vi "Run - TDMS Logging (SubVI).vi"(8 "error in (no error)":errorcluster, 10 "Cluster":T1={"Test Plan"=[], "PlanRow"=0, "Device Name"=[], "Timeout"=0, "Start?"=FALSE, "Pause?"=FALSE, "IP Address"=[], "LogRow"=0, "Logtype"=0, "Log Elapse"=0.0, "Data"={"Station"="", "Sample ID"="", "Job No"="", "Job Description"="", "Path"=path "", "Delay"=timestamp(-28800 s since 1904-01-01), "Square"=FALSE, "Test Type"=0, "Speciment No"="", "Depth"="", "Height"="", "Diameter/Length"="", "Weight"=""}, "Stop log?"=FALSE, "tdms"=refnum, "Sensor Data"=[], "Start time"=timestamp(0 s since 1904-01-01), "Prev Log Elapse"=0, "Plot"=0, "X-Axis"=[], "Y-Axis"=[], "XY"=[], "End Stage?"=FALSE, "1run"=FALSE, "Condition"=[], "Start Con"=FALSE, "Log Con"=FALSE, "Stop Con"=FALSE, "Start Elapse"=0.0, "Start Load"=0.0, "Motor"=0, "StartRow"=0, "number log"=0, "Dir"=FALSE, "Start time test"=timestamp(0 s since 1904-01-01), "Auto"=FALSE, "Check return?"=FALSE, "Inv"={"M"=[], "Bool"=[]}, "tdms temp"=refnum, "Zero?"=FALSE, "Graph timer"=0.0, "Square"=FALSE, "Plot Timer"=0.0, "1st Run"=FALSE, "TDMS Path"=path "", "MaxLoad"=0.0, "Log Timer"=[], "Test Type"=0, "Log Sensor"=[], "Save?"=FALSE, "1st Log"=FALSE, "Y-Axis 2"=[], "On Y-Axis 2"=FALSE, "Decimal"=[], "Init"={"PWP"=0.0, "Load"=0.0, "Volume"=0.0, "Disp"=0.0, "CP"=0.0, "Vol In"=0.0, "Vol Out"=0.0}, "Calc"={"TS"={"Change PWP"=0.0, "Change Vol"=0.0, "Axial Load"=0.0, "CiL"=0.0, "Deviator"=0.0, "Axial Strain"=0.0}, "TUU"={"Change PWP"=0.0, "Axial Load"=0.0, "CiL"=0.0, "Deviator"=0.0, "Axial Strain"=0.0}, "Sat"={"Change PWP"=0.0, "Volume Change"=0.0, "B Value"=0.0, "PWP Diss"=0.0}, "Per"={"Change Vol In"=0.0, "Change Vol Out"=0.0, "Mean Vol"=0.0}, "Step Cons"={"V Stress"=0.0, "H Settlement"=0.0}, "UCT"={"ALC"=0.0, "H Change"=0.0, "Deviator"=0.0, "Axial Strain"=0.0}}, "Device Index"=[], "Channel Index"=[], "http ref"=refnum} {"Test Type" items=["Please Select", "Triaxial Shear", "Triaxial UU", "Shearbox", "Permeability", "Consolidation", "Saturation", "User Defined"]; "Data"."Test Type" items=["Please Select", "Triaxial Shear", "Triaxial UU", "Shearbox", "Permeability", "Consolidation", "Saturation", "User Defined"]; "Data"."Delay" format="%<%H:%M:%S>T"}) -> (0 "error out":errorcluster)   [LabVIEW 2019]
uses:
  Controls/RunTest - Data Structure.ctl
  Controls/Test Panel - Data Structure.ctl
  Controls/Station - Test Type.ctl
  Controls/RunTest - Calculate Data.ctl
  <vilib>/httpClient/ClientHandle.ctl
  <vilib>/httpClient/LabVIEWHTTPClient.lvlib
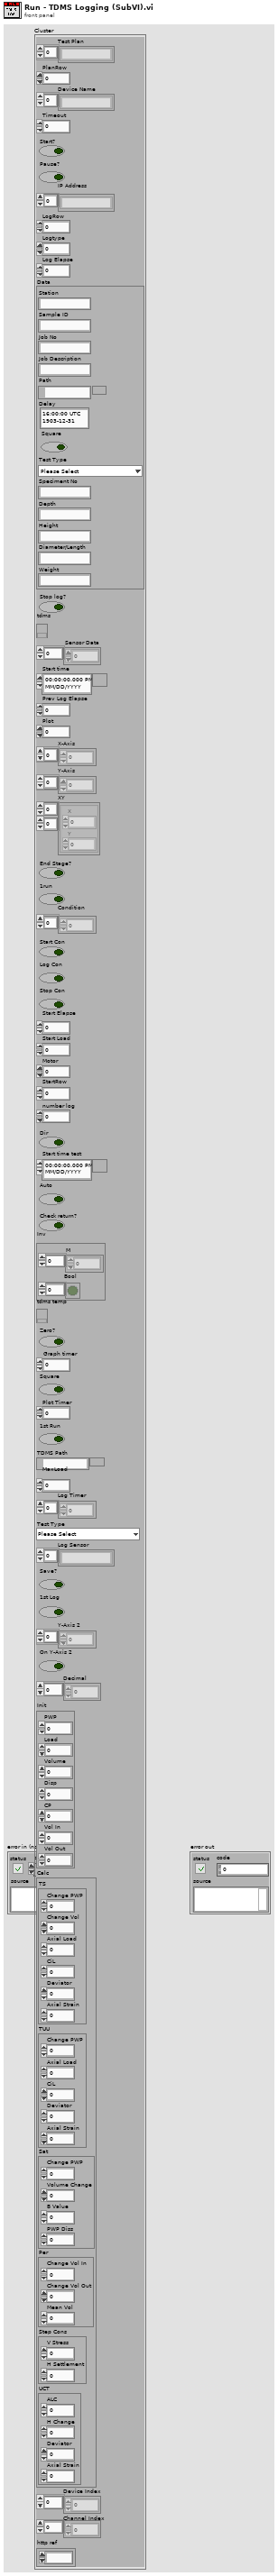
[diagram p1: front panel]
types:
  T1 = typedef "RunTest - Data Structure.ctl" = cluster{"Test Plan":string[], "PlanRow":i32, "Device Name":string[], "Timeout":i32, "Start?":bool, "Pause?":bool, "IP Address":string[], "LogRow":i32, "Logtype":u16, "Log Elapse":sgl, "Data":T2, "Stop log?":bool, "tdms":refnum<k34>, "Sensor Data":sgl[], "Start time":timestamp, "Prev Log Elapse":u32, "Plot":u16, "X-Axis":u16[], "Y-Axis":u16[], "XY":cluster{"X":dbl, "Y":dbl}[][], "End Stage?":bool, "1run":bool, "Condition":u16[], "Start Con":bool, "Log Con":bool, "Stop Con":bool, "Start Elapse":dbl, "Start Load":dbl, "Motor":i32, "StartRow":i32, "number log":i32, "Dir":bool, "Start time test":timestamp, "Auto":bool, "Check return?":bool, "Inv":cluster{"M":i32[], "Bool":bool[]}, "tdms temp":refnum<k34>, "Zero?":bool, "Graph timer":dbl, "Square":bool, "Plot Timer":dbl, "1st Run":bool, "TDMS Path":path, "MaxLoad":dbl, "Log Timer":sgl[], "Test Type":T3, "Log Sensor":string[], "Save?":bool, "1st Log":bool, "Y-Axis 2":u16[], "On Y-Axis 2":bool, "Decimal":u8[], "Init":cluster{"PWP":sgl, "Load":sgl, "Volume":sgl, "Disp":sgl, "CP":sgl, "Vol In":sgl, "Vol Out":sgl}, "Calc":T4, "Device Index":i32[], "Channel Index":i32[], "http ref":T5}
  T2 = typedef "Test Panel - Data Structure.ctl" = cluster{"Station":string, "Sample ID":string, "Job No":string, "Job Description":string, "Path":path, "Delay":timestamp, "Square":bool, "Test Type":T3, "Speciment No":string, "Depth":string, "Height":string, "Diameter/Length":string, "Weight":string}
  T3 = typedef "Station - Test Type.ctl" = u16
  T4 = typedef "RunTest - Calculate Data.ctl" = cluster{"TS":cluster{"Change PWP":sgl, "Change Vol":sgl, "Axial Load":sgl, "CiL":sgl, "Deviator":sgl, "Axial Strain":sgl}, "TUU":cluster{"Change PWP":sgl, "Axial Load":sgl, "CiL":sgl, "Deviator":sgl, "Axial Strain":sgl}, "Sat":cluster{"Change PWP":sgl, "Volume Change":sgl, "B Value":sgl, "PWP Diss":sgl}, "Per":cluster{"Change Vol In":sgl, "Change Vol Out":sgl, "Mean Vol":sgl}, "Step Cons":cluster{"V Stress":sgl, "H Settlement":sgl}, "UCT":cluster{"ALC":sgl, "H Change":sgl, "Deviator":sgl, "Axial Strain":sgl}}
  T5 = typedef "LabVIEWHTTPClient.lvlib/ClientHandle.ctl" = refnum<k1>
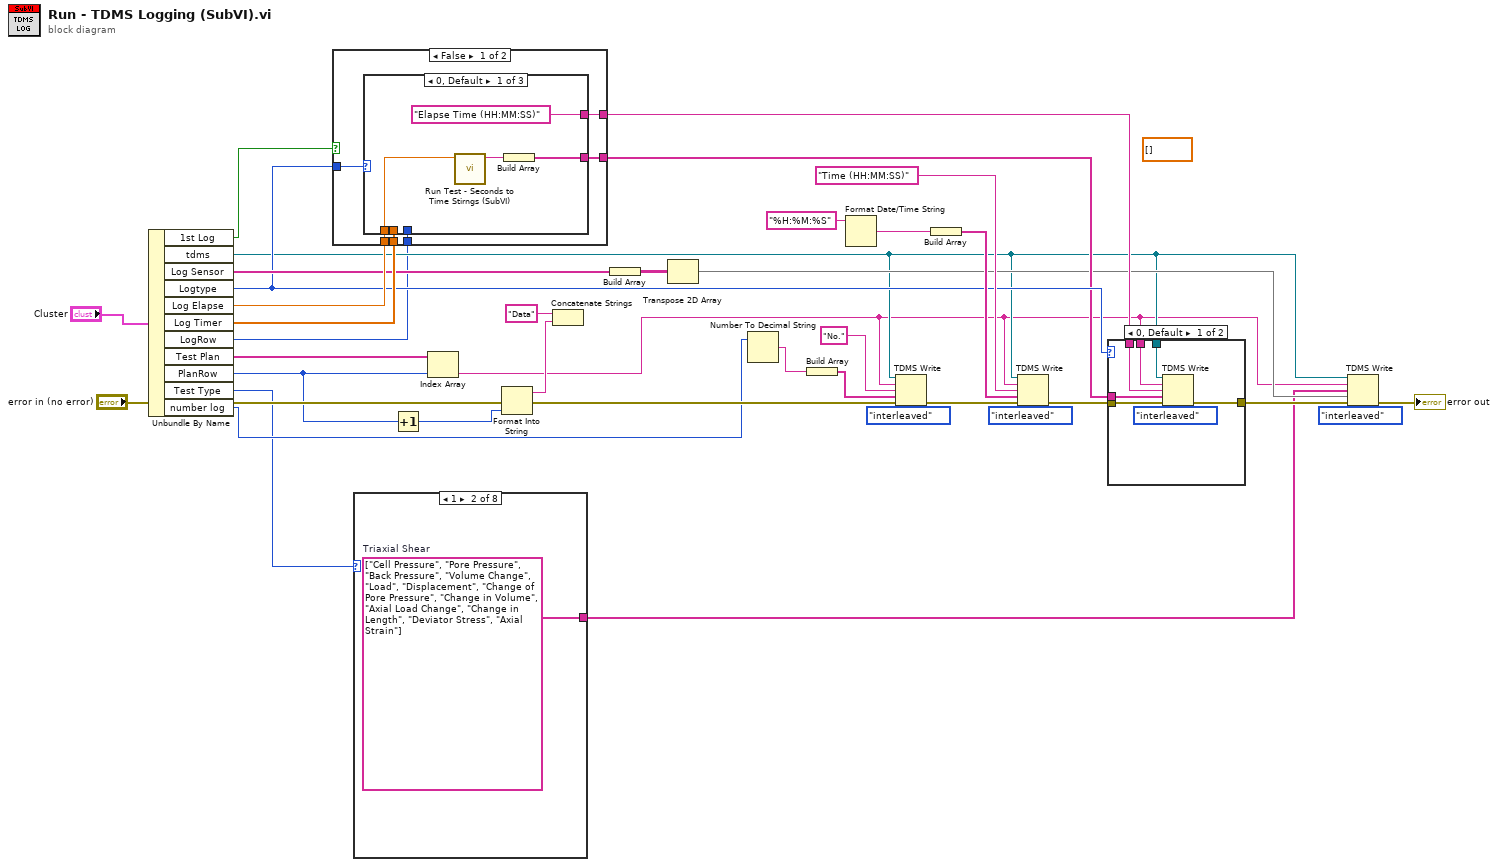
[diagram p0: block diagram]
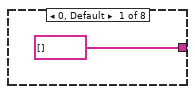
[diagram p2: hidden frame]
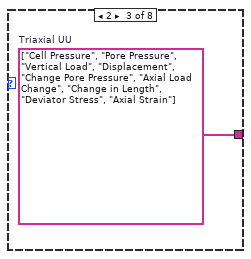
[diagram p3: hidden frame]
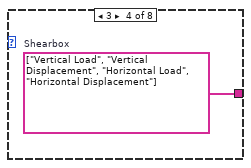
[diagram p4: hidden frame]
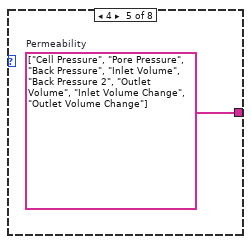
[diagram p5: hidden frame]
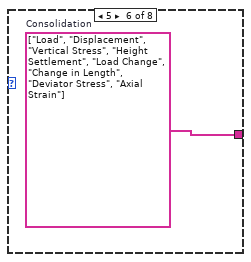
[diagram p6: hidden frame]
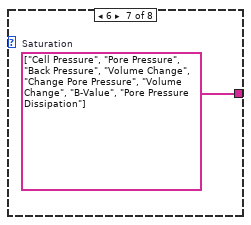
[diagram p7: hidden frame]
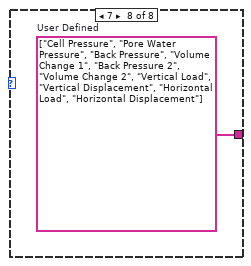
[diagram p8: hidden frame]
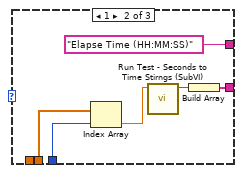
[diagram p9: hidden frame]
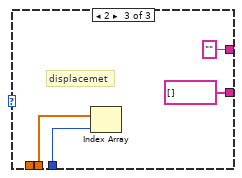
[diagram p10: hidden frame]
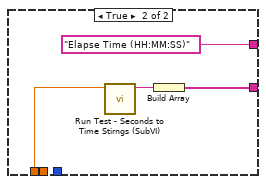
[diagram p11: hidden frame]
diagram:
  (unwired) dbl[] [] ("Sensor Data")
  n1 = Unbundle By Name("Cluster") -> ("1st Log"=w15:bool, "tdms"=w11:refnum<k34>, "Log Sensor"=w27:string[], "Logtype"=w20:u16, "Log Elapse"=w29:sgl, "Log Timer"=w30:sgl[], "LogRow"=w7:i32, "Test Plan"=w6:string[], "PlanRow"=w5:i32, "Test Type"=w2:T3, "number log"=w3:i32)
  n2 = case shown="False" w15 {
    tunnel: w30 -> [w43 _]
    tunnel: w7 -> [w42 _]
    tunnel: w29 -> [w41 w61]
    tunnel: w20 -> [w40 _]
    tunnel: [w39 "Elapse Time (HH:MM:SS)" ("String")] -> w19
    tunnel: [w38 w59] -> w18
    frame False {
      n3 = case shown="0, Default" w40 {
        tunnel: w43 -> [_ w53 w57]
        tunnel: w42 -> [_ w52 w56]
        tunnel: w41 -> [w45 _ _]
        tunnel: ["Elapse Time (HH:MM:SS)" ("String") "Elapse Time (HH:MM:SS)" ("String") "" ("String")] -> w39
        tunnel: [w46 w49 string[] []] -> w38
        frame 0, Default {
          n4 = call "Run Test - Seconds to Time Stirngs (SubVI).vi"("Seconds"=w45) -> ("Time Strings"=w44:string)  [unwired: 10 in]
          n5 = Build Array(w44) -> (w46:string[])
        }
        frame 1 {
          n6 = Index Array(array=w53, index=w52) -> (element=w48:sgl)
          n7 = call "Run Test - Seconds to Time Stirngs (SubVI).vi"("Seconds"=w48) -> ("Time Strings"=w51:string)  [unwired: 10 in]
          n8 = Build Array(w51) -> (w49:string[])
        }
        frame 2 {
          # "displacemet"
          n9 = Index Array(array=w57, index=w56) -> ()  [unwired: 1 out]
        }
      }
    }
    frame True {
      n10 = call "Run Test - Seconds to Time Stirngs (SubVI).vi"("Seconds"=w61) -> ("Time Strings"=w58:string)  [unwired: 10 in]
      n11 = Build Array(w58) -> (w59:string[])
    }
  }
  n12 = case shown="1" w2 {
    tunnel: [string[] [] w63 w64 w65 w66 w67 w68 w69] -> w1
    frame 0, Default {
    }
    frame 1 {
      w63 = string[] ["Cell Pressure", "Pore Pressure", "Back Pressure", "Volume Change", "Load", "Displacement", "Change of Pore Pressure", "Change in Volume", "Axial Load Change", "Change in Length", "Deviator Stress", "Axial Strain"]  # Triaxial Shear
    }
    frame 2 {
      w64 = string[] ["Cell Pressure", "Pore Pressure", "Vertical Load", "Displacement", "Change Pore Pressure", "Axial Load Change", "Change in Length", "Deviator Stress", "Axial Strain"]  # Triaxial UU
    }
    frame 3 {
      w65 = string[] ["Vertical Load", "Vertical Displacement", "Horizontal Load", "Horizontal Displacement"]  # Shearbox
    }
    frame 4 {
      w66 = string[] ["Cell Pressure", "Pore Pressure", "Back Pressure", "Inlet Volume", "Back Pressure 2", "Outlet Volume", "Inlet Volume Change", "Outlet Volume Change"]  # Permeability
    }
    frame 5 {
      w67 = string[] ["Load", "Displacement", "Vertical Stress", "Height Settlement", "Load Change", "Change in Length", "Deviator Stress", "Axial Strain"]  # Consolidation
    }
    frame 6 {
      w68 = string[] ["Cell Pressure", "Pore Pressure", "Back Pressure", "Volume Change", "Change Pore Pressure", "Volume Change", "B-Value", "Pore Pressure Dissipation"]  # Saturation
    }
    frame 7 {
      w69 = string[] ["Cell Pressure", "Pore Water Pressure", "Back Pressure", "Volume Change 1", "Back Pressure 2", "Volume Change 2", "Vertical Load", "Vertical Displacement", "Horizontal Load", "Horizontal Displacement"]  # User Defined
    }
  }
  n13 = Increment(x=w5) -> (x+1=w34:i32)
  n14 = Index Array(array=w6, index=w5) -> (element=w4:string)
  n15 = Format Into String(error in="error in (no error)", w34) -> (resulting string=w37:string, error out=w13:errorcluster)  [unwired: 2 in]
  n16 = Concatenate Strings("Data" ("group name in (Untitled)"), w37) -> ()  [unwired: 1 out]
  n17 = Build Array(w27) -> (w17:string[][])
  n18 = Transpose 2D Array(2D array=w17) -> (transposed array=w16:string[][])
  n19 = Number To Decimal String(number=w3) -> (decimal integer string=w9:string)  [unwired: 1 in]
  n20 = Build Array(w9) -> (w8:string[])
  n21 = Format Date/Time String(time format string (%c)="%H:%M:%S") -> (date/time string=w24:string)  [unwired: 2 in]
  n22 = TDMS Write(0:w11, 1:enum16{"decimated", "interleaved"}."interleaved" ("data layout (0:decimated)"), 5:w4, 7:"No." ("String"), 9:w8, 11:w13) -> (15:w12:errorcluster)  [unwired: 3 out]
  n23 = Build Array(w24) -> (w26:string[])
  n24 = TDMS Write(0:w11, 1:enum16{"decimated", "interleaved"}."interleaved" ("data layout (0:decimated)"), 5:w4, 7:"Time (HH:MM:SS)" ("String"), 9:w26, 11:w12) -> (15:w22:errorcluster)  [unwired: 3 out]
  n25 = case shown="0, Default" w20 {
    tunnel: w22 -> [w75 w77]
    tunnel: [w74 w77] -> w21
    tunnel: w11 -> [w73 _]
    tunnel: w4 -> [w72 _]
    tunnel: w19 -> [w71 _]
    tunnel: w18 -> [w70 _]
    frame 0, Default {
      n26 = TDMS Write(0:w73, 1:enum16{"decimated", "interleaved"}."interleaved" ("data layout (0:decimated)"), 5:w72, 7:w71, 9:w70, 11:w75) -> (15:w74:errorcluster)  [unwired: 3 out]
    }
    frame 2 {
    }
  }
  n27 = TDMS Write(0:w11, 1:enum16{"decimated", "interleaved"}."interleaved" ("data layout (0:decimated)"), 5:w4, 7:w1, 9:w16, 11:w21) -> (15:→"error out":errorcluster)  [unwired: 3 out]
